vi "Get Visible Items.vi"(8 "error in":errorcluster, 11 "TreeControl in":refnum<vi>) -> (0 "error out":errorcluster, 2 "Visible Item Tags":string[](array[string]), 3 "TreeControl out":refnum<vi>)   [LabVIEW 2013, in "LVTM.lvlib"]
uses:
  LVTM.lvlib
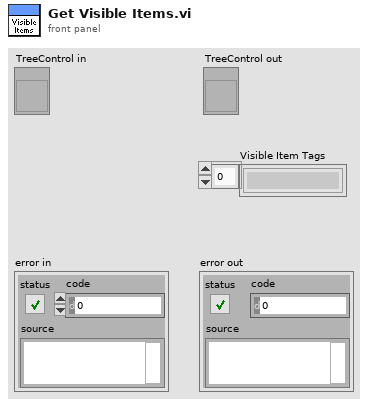
[diagram p1: front panel]
types:
  T1 = typedef "LVNodeAndColumnTypeDef.ctl" = cluster{"Node":string, "Column":i32}
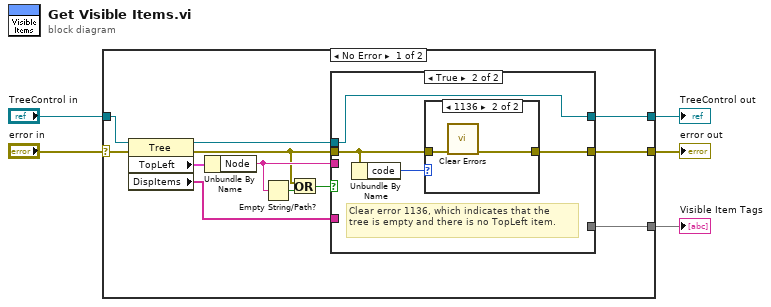
[diagram p0: block diagram]
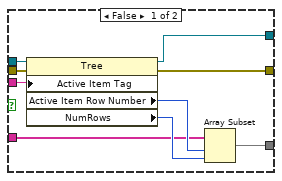
[diagram p2: hidden frame]
diagram:
  n1 = case shown="No Error" "error in" {
    selector: "error in" -> [w8 w34]
    tunnel: [w17 w34] -> w5
    tunnel: [w16 _] -> w4
    tunnel: [w13 w35] -> w3
    tunnel: "TreeControl in" -> [w12 w35]
    frame No Error {
      n2 = property on="Property Node" class="Tree"(reference=w12, error in=w8) -> (reference out=w11:refnum<vi>, error out=w6:errorcluster, "TopLeft"=w14:T1, "DispItems"=w15:string[])
      n3 = Unbundle By Name(w14) -> ("Node"=w9:string)
      n4 = Empty String/Path?(string/path=w9) -> (empty?=w10:bool)
      n5 = Or(x=w6, y=w10) -> (x .or. y?=w7:bool)
      n6 = case shown="True" w7 {
        tunnel: [w26 w29] -> w17
        tunnel: [w24 _] -> w16
        tunnel: w15 -> [w22 _]
        tunnel: w9 -> [w21 _]
        tunnel: [w20 w30] -> w13
        tunnel: w11 -> [w19 w30]
        tunnel: w6 -> [w18 w28]
        frame False {
          n7 = property on="Property Node" class="Tree"(reference=w19, error in=w18, "Active Item Tag"=w21) -> (reference out=w20:refnum<vi>, error out=w26:errorcluster, "Active Item Row Number"=w23:i32, "NumRows"=w25:u32)
          n8 = Array Subset(array=w22, index=w23, length=w25) -> (w24:string[])
        }
        frame True {
          # "Clear error 1136, which indicates that the\ntree is empty and there is no TopLeft item."
          n9 = Unbundle By Name(w28) -> ("code"=w27:i32)
          n10 = case shown="1136" w27 {
            tunnel: [w31 w33] -> w29
            tunnel: w28 -> [w31 w32]
            frame 0, Default {
            }
            frame 1136 {
              n11 = call <vilib>:"Clear Errors.vi"("error in (no error)"=w32) -> ("error out"=w33:errorcluster)  [unwired: 6 in]
            }
          }
        }
      }
    }
    frame Error {
    }
  }
  "error out" <- w5
  "Visible Item Tags" <- w4
  "TreeControl out" <- w3
